vi "MCL Trigger Waveform Acquisition.vi"(7 "handle":i32, 9 "waveform":dbl, 10 "DataPoints":u32, 11 "axis":u32) -> (1 "waveform out":dbl, 3 "function return":i32)   [LabVIEW 2017, in "Madlib.lvlib"]
doc: "MADLIB_API int MCL_TriggerWaveformAcquisition(unsigned int axis, unsigned int DataPoints, double* waveform, int handle);"
uses:
  Madlib.lvlib
  Madlib.dll
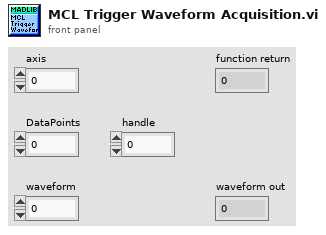
[diagram p1: front panel]
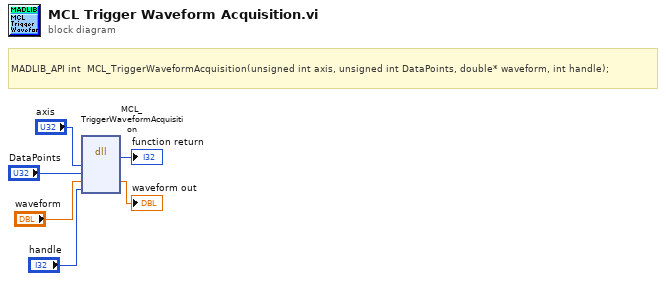
[diagram p0: block diagram]
diagram:
  # "MADLIB_API\tint\t\tMCL_TriggerWaveformAcquisition(unsigned int axis, unsigned int DataPoints, double* waveform, int handle);"
  n1 = dll-call lib="C:/Users/francesco/dev/pump-probe/Piezo/lvlib/Madlib.*" fn="MCL_TriggerWaveformAcquisition"("axis"="axis", "DataPoints"="DataPoints", "waveform"="waveform", "handle"="handle") -> (→"function return":i32, "waveform"=→"waveform out":dbl)  [unwired: 6 in, 2 out]
